vi "controlChainGain.vi"(7 "Set":bool, 8 "error in":errorcluster, 9 "attenuation [0...3]":i32, 10 "axis in":u8, 11 "connection ID":refnum<k5>) -> (0 "error out":errorcluster, 1 "attenuation out":i32, 2 "axis out":i32, 3 "connection ID":refnum<k5>)   [LabVIEW 2016, in "AMC_VIs.lvlib"]
doc: "Retrieves or sets the signal chain gain to control overall power. The attenuation can be chosen as follows:\n0: 0 dB attenuation\n1: 10 dB attenuation\n2: 15 dB attenuation\n3: 20 dB attenuation"
uses:
  AMC_VIs.lvlib
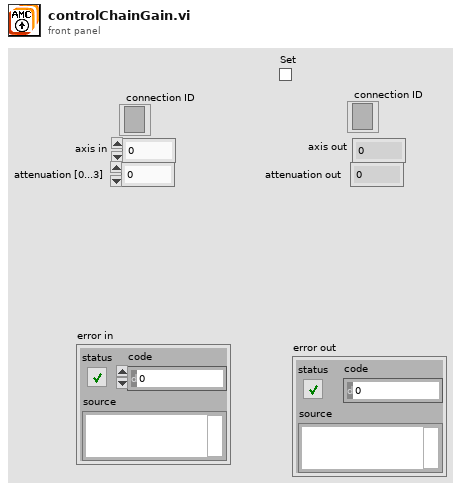
[diagram p1: front panel]
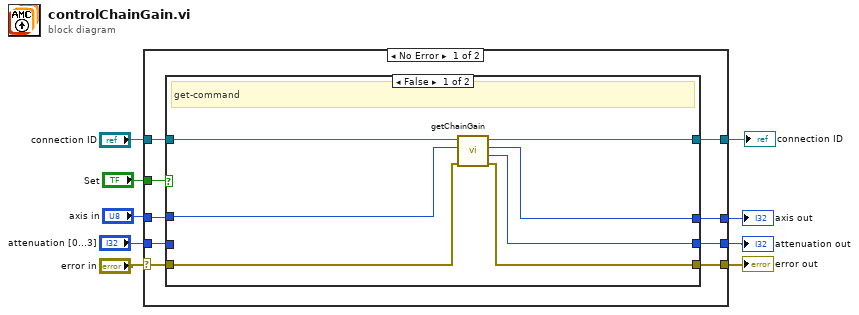
[diagram p0: block diagram]
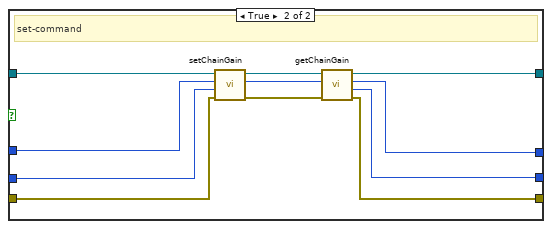
[diagram p2: hidden frame]
diagram:
  n1 = case shown="No Error" "error in" {
    selector: "error in" -> [w14 w40]
    tunnel: "axis in" -> [w18 w37]
    tunnel: [w10 w40] -> w8
    tunnel: "attenuation [0...3]" -> [w16 w38]
    tunnel: [w13 w38] -> w3
    tunnel: "Set" -> [w15 _]
    tunnel: [w12 w39] -> w6
    tunnel: "connection ID" -> [w17 w39]
    tunnel: [w11 w37] -> w1
    frame No Error {
      n2 = case shown="False" w15 {
        tunnel: w17 -> [w23 w36]
        tunnel: w18 -> [w24 w32]
        tunnel: w16 -> [_ w27]
        tunnel: w14 -> [w25 w33]
        tunnel: [w19 w26] -> w13
        tunnel: [w22 w34] -> w12
        tunnel: [w21 w29] -> w11
        tunnel: [w20 w28] -> w10
        frame False {
          # "get-command"
          n3 = call "getChainGain.vi"("error in"=w25, "axis"=w24, "connection ID"=w23) -> ("error out"=w20:errorcluster, "gaincoeff"=w19:i32, "axis_out"=w21:i32, "connection ID"=w22:refnum<k5>)  [unwired: 5 in]
        }
        frame True {
          # "set-command"
          n4 = call "setChainGain.vi"("error in"=w33, "gainconfig"=w27, "axis"=w32, "connection ID"=w36) -> ("error out"=w31:errorcluster, "axis_out"=w30:i32, "connection ID"=w35:refnum<k5>)  [unwired: 5 in]
          n5 = call "getChainGain.vi"("error in"=w31, "axis"=w30, "connection ID"=w35) -> ("error out"=w28:errorcluster, "gaincoeff"=w26:i32, "axis_out"=w29:i32, "connection ID"=w34:refnum<k5>)  [unwired: 5 in]
        }
      }
    }
    frame Error {
    }
  }
  "error out" <- w8
  "axis out" <- w1
  "attenuation out" <- w3
  "connection ID" <- w6
